vi "CLUSTER.vi"(0 "MIN SIZE":i32=4, 4 "MAX SIZE":i32=300, 6 "유클리디언":dbl, 10 "array with duplicates removed":i32[][](array[numeric])) -> (3 "Array":cluster{i32[], i32[]}[](array[cluster]))   [LabVIEW 2023]
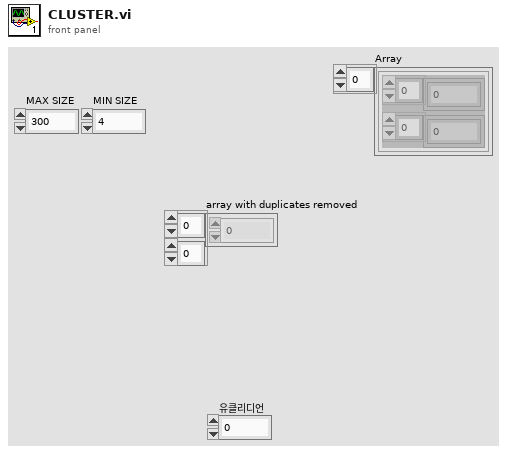
[diagram p1: front panel]
types:
  T1 = cluster{"array with duplicates removed":i32[], "array with duplicates removed":i32[]}
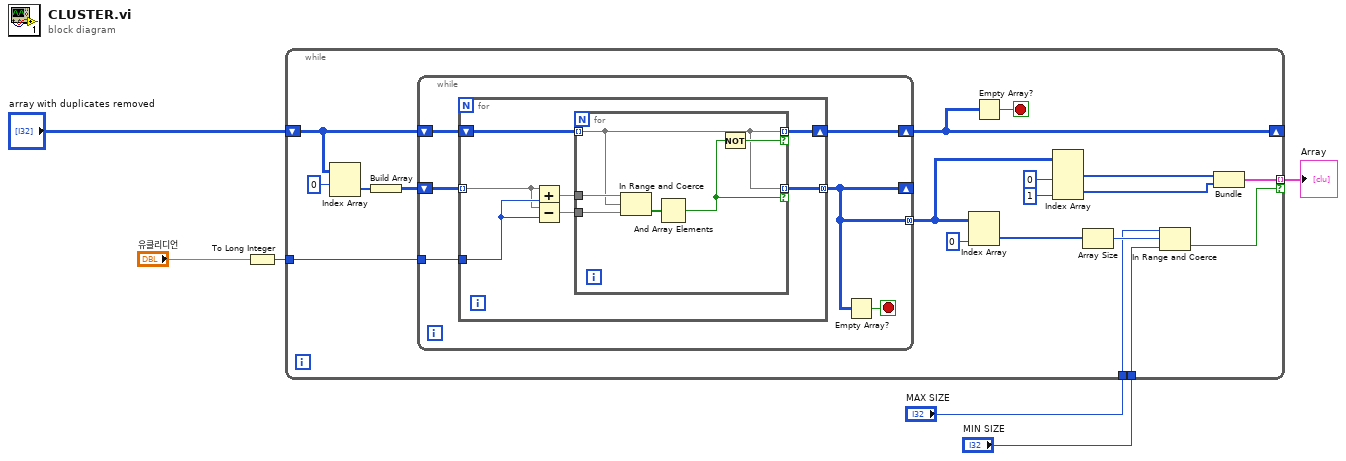
[diagram p0: block diagram]
diagram:
  n1 = To Long Integer(number="유클리디언") -> (32bit integer=w5:i32)
  n2 = while {
    shift-right: [w19] -> _
    shift-left: "array with duplicates removed" -> [w23]
    tunnel: w5 -> [w21]
    tunnel: [w20] -> w4 mode=indexing if=w9
    tunnel: "MIN SIZE" -> [w16]
    tunnel: "MAX SIZE" -> [w10]
    stop <- w18 stop-if-true
    n3 = Index Array(array=w23, index (row)=0 ("index")) -> (element=w24:i32[])  [unwired: 1 in]
    n4 = Build Array(w24) -> (w22:i32[][])
    n5 = while {
      shift-right: [w30] -> w19
      shift-left: w23 -> [w31]
      shift-right: [w26] -> _
      shift-left: w22 -> [w29]
      tunnel: w21 -> [w28]
      tunnel: [w26] -> w15 mode=concatenating
      stop <- w27 stop-if-true
      n6 = for {
        shift-right: [w37] -> w30
        shift-left: w31 -> [w38]
        tunnel: w29 -> [w32] mode=indexing
        tunnel: w28 -> [w33]
        tunnel: [w34] -> w26 mode=concatenating
        n7 = Add(x=w32, y=w33) -> (x+y=w36:i32[])
        n8 = Subtract(x=w32, y=w33) -> (x-y=w35:i32[])
        n9 = for {
          tunnel: w38 -> [w39] mode=indexing
          tunnel: [w39] -> w37 mode=indexing if=w42
          tunnel: w36 -> [w44]
          tunnel: w35 -> [w43]
          tunnel: [w39] -> w34 mode=indexing if=w40
          n10 = In Range and Coerce(upper limit=w44, x=w39, lower limit=w43) -> (In Range?=w41:bool[])  [unwired: 1 out]
          n11 = And Array Elements(Boolean array=w41) -> (logical AND=w40:bool)
          n12 = Not(x=w40) -> (.not. x?=w42:bool)
        }
      }
      n13 = Empty Array?(array=w26) -> (empty?=w27:bool)
    }
    n14 = Index Array(array=w15, index (col)=0 ("비활성화된 인덱스 (열)")) -> (element=w12:i32[])  [unwired: 1 in]
    n15 = Empty Array?(array=w19) -> (empty?=w18:bool)
    n16 = Index Array(array=w15, index (col) #1=0 ("인덱스 (행)"), index (col) #2=1 ("인덱스 (행)")) -> (element #1=w8:i32[], element #2=w7:i32[])  [unwired: 2 in]
    n17 = Array Size(array=w12) -> (size(s)=w11:i32)
    n18 = In Range and Coerce(upper limit=w10, x=w11, lower limit=w16) -> (In Range?=w9:bool)  [unwired: 1 out]
    n19 = Bundle("array with duplicates removed"=w8, "array with duplicates removed"=w7) -> (w20:T1)  [unwired: 1 in]
  }
  "Array" <- w4
